vi "Initial Target Angle Immediate.vi"(10 "Target Real Angle":dbl) -> ()   [LabVIEW 2019]
uses:
  Framework/Robot Global Data.vi
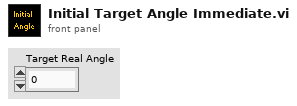
[diagram p1: front panel]
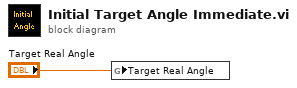
[diagram p0: block diagram]
diagram:
  n1 = global write "Robot Global Data.vi" "Target Real Angle"("Target Real Angle") -> ()
